vi "PredefinedSplit.vi"(6 "Groups":string[][](array[string]), 8 "error in (no error)":errorcluster caption="entrée d'erreur (pas d'erreur)", 9 "y":string[][](array[string]), 10 "X":string[][](array[string]), 11 "PredefinedSplit":cluster{"test_fold":dbl[]}) -> (0 "error out":errorcluster caption="sortie d'erreur", 3 "Split":T1(array[cluster]))   [LabVIEW 2020]
doc: "Predefined split cross-validator\n\nProvides train/test indices to split data into train/test sets using a predefined scheme specified by the user with the test_fold parameter.\n\n\nParameters :\n\n- test_fold : array-like of shape (n_samples,)\nThe entry test_fold[i] represents the index of the test set that sample i belongs to. It is possible to exclude sample i from any test set (i.e. include sample i in every training set) by setting test_fold[i] equal to -1.\n\n\n\nMethods : Split\n\n\nGenerate indices to split data into training and test set.\n\nParameters :\n\n- X : object\nAlways ignored, exists for compatibility.\n\n- y : object\nAlways ignored, exists for compatibility.\n\n- group : sobject\nAlways ignored, exists for compatibility.\n\nYields : \n\n- train : ndarray\nThe training set indices for that split.\n\n- test : ndarray\nThe testing set indices for that split."
uses:
  PredefinedSplit.lvclass
panel:
  out "PredefinedSplit.lvclass":refnum<class "PredefinedSplit.lvclass">
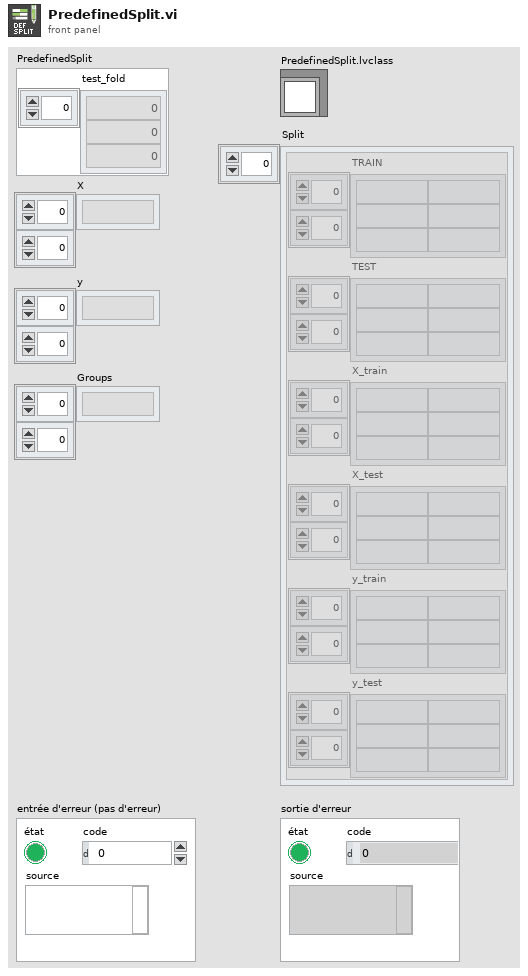
[diagram p1: front panel]
types:
  T1 = cluster{"TRAIN":string[][], "TEST":string[][], "X_train":string[][], "X_test":string[][], "y_train":string[][], "y_test":string[][]}[]
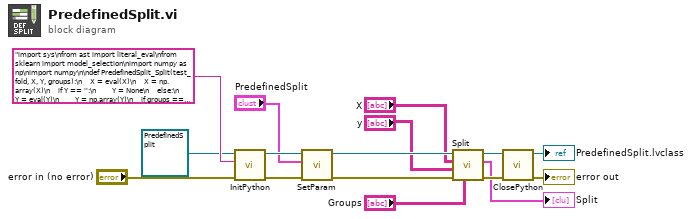
[diagram p0: block diagram]
diagram:
  n1 = call-dynamic "InitPython.vi"("error in (no error)"="error in (no error)", "Python Instruction"="import sys\nfrom ast import literal_eval\nfrom sklearn import model_selection\nimport numpy as np\nimport numpy\n\ndef PredefinedSplit_Split(test_fold, X, Y, groups):\n    X = eval(X)\n    X = np.array(X)\n    if Y == '':\n        Y = None\n    else:\n        Y = eval(Y)\n        Y = np.array(Y)\n    if groups == '':\n        groups = None\n    else:\n        groups = eval(groups)\n        groups = np.array(groups)\n    list_return = []\n    try:\n        for train_index, test_index in model_selection.PredefinedSplit(test_fold).split(X, Y, groups):\n            list_return = list_return +[\"TRAIN:\", train_index.tolist(), \"TEST:\", test_index.tolist()]\n            X_train, X_test = X[train_index].tolist(), X[test_index].tolist()\n            y_train, y_test = Y[train_index].tolist(), Y[test_index].tolist()\n            list_return = list_return +[\"X_train:\", X_train, \"X_test:\", X_test, \"y_train:\", y_train, \"y_test:\", y_test]\n        return str(list_return)\n    except:\n        erreur = sys.exc_info()\n        typerr = u\"%s\" % (erreur[0])\n        typerr = typerr[typerr.find(\"'\")+1:typerr.rfind(\"'\")]\n        msgerr = u\"%s\" % (erreur[1])\n        message = str('/!\\\\ {0} : {1}'. format(typerr,msgerr))\n        return message", "Scikit-learn en entrée"=refnum<class "PredefinedSplit.lvclass"> refnum ("PredefinedSplit.lvclass")) -> ("error out"=w14:errorcluster, "Scikit-learn en sortie"=w13:refnum<class "PredefinedSplit.lvclass">)  [unwired: 7 in]
  n2 = call-dynamic "SetParam.vi"("error in (no error)"=w14, "PredefinedSplit"="PredefinedSplit", "PredefinedSplit.lvclass"=w13) -> ("error out"=w10:errorcluster, "PredefinedSplit.lvclass"=w9:refnum<class "PredefinedSplit.lvclass">)  [unwired: 7 in]
  n3 = call-dynamic "Split.vi"("Groups"="Groups", "error in (no error)"=w10, "y"="y", "X"="X", "PredefinedSplit.lvclass"=w9) -> ("error out"=w8:errorcluster, "Split"=→"Split":T1, "PredefinedSplit.lvclass"=w7:refnum<class "PredefinedSplit.lvclass">)  [unwired: 4 in]
  n4 = call-dynamic "ClosePython.vi"("error in (no error)"=w8, "Scikit-learn en entrée"=w7) -> ("error out"=→"error out":errorcluster, "Scikit-learn en sortie"=→"PredefinedSplit.lvclass":refnum<class "PredefinedSplit.lvclass">)  [unwired: 8 in]
